vi "Sample_Finite_HardwareDelay.vi"() -> ()   [LabVIEW 2013]
doc: "This samples demonstrates how to sample a finite waveform."
uses:
  <userlib>/ArtScope/Trigger/ArtScope_ConfigureTriggerDigital.vi
  <userlib>/ArtScope/Fetch/ArtScope_FetchBinary16.vi
  <userlib>/ArtScope/_SubVI/ArtScope_ArrayByChannel_U16.vi
panel:
  out "error out":errorcluster
  in  "reference position":dbl
  in  "source":string(combo)="VAL_TRIGGER_DTR"
  in  "edge":i32(ring) items=["Negative", "Positive", "NegatiPosit"]
  in  "sensitive":i32=50
  in  "count":i32=1
  in  "range(Vpp)":i32(ring)=1 items=["20V", "10V", "2V", "40V", "16V", "8V", "4V", "1.6V", "800m", "400m", "160m", "80m", "40m"]
  in  "offset(mV)":i32
  in  "NumSamples":i32=1000
  in  "Stop":bool
  out "waveform":u16[][](graph)
  in  "Timeout(s)":dbl=10.0
  in  "MinRecordLength":i32=6000
  in  "MinSampleRate":dbl=800000.0
  in  "Coupling":i32(ring) items=["DC", "AC"]
  in  "Channel Name":string="0,1"
  in  "Resource Name":string="Dev1"
  # "Vertical"
  # "Horizontal"
  # "Trigger"
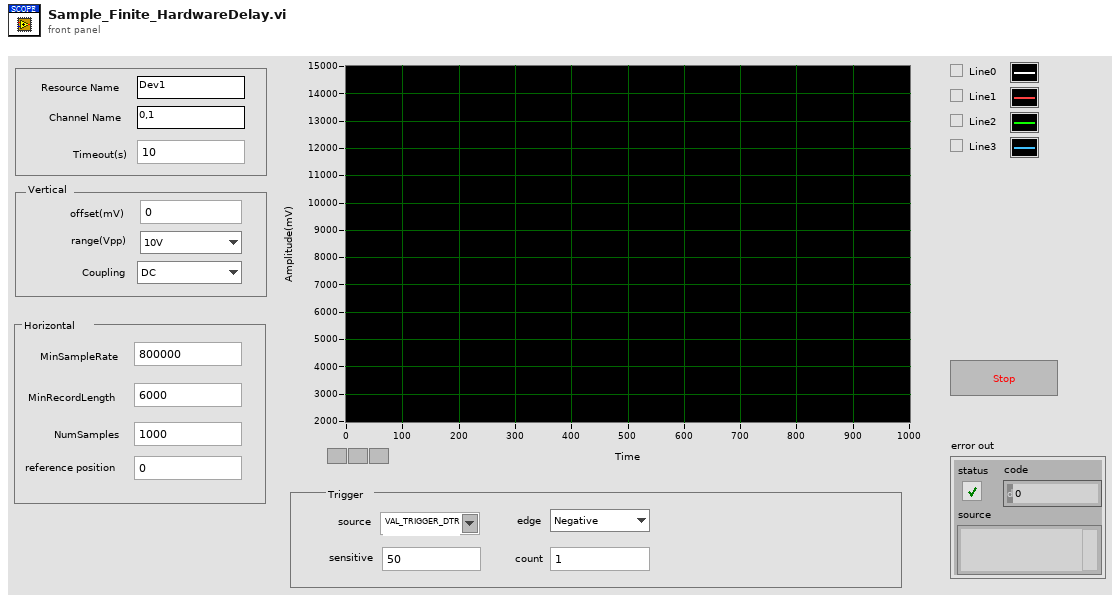
[diagram p1: front panel]
types:
  T1 = cluster{"fLSB":cluster{dbl, dbl, dbl, dbl, dbl, dbl, dbl, dbl}, "RangeValue":cluster{dbl, dbl, dbl, dbl, dbl, dbl, dbl, dbl}, "wMaxLSB":u32, "TriggerMode":i32, "sampLengthPerChan":u32, "pAvailSampsPoints":u32, "channelCount":i32}
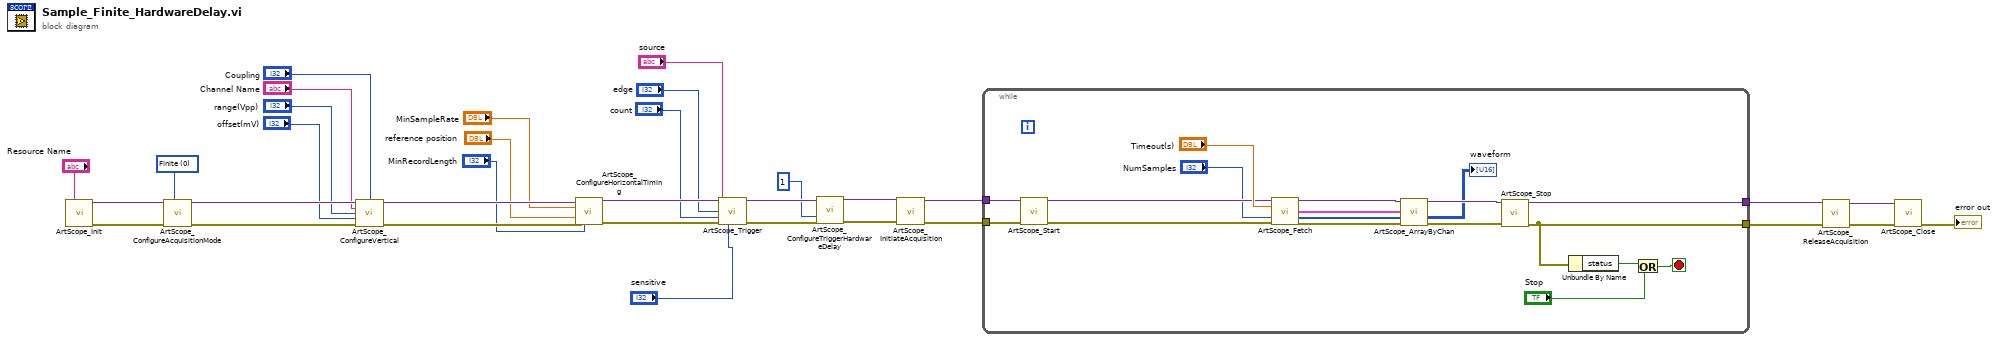
[diagram p0: block diagram]
diagram:
  w26 = 0 items=["Finite", "Continuous"] ("AcuqMode")
  n1 = call <userlib>:"ArtScope_Init.vi"("task name"="Resource Name") -> ("task handle"=w27:variant, "error out"=w28:errorcluster)  [unwired: 13 in]
  n2 = call <userlib>:"ArtScope_ConfigureAcquisitionMode.vi"("task handle"=w27, "acquisition mode"=w26, "error in (no error)"=w28) -> ("task handle"=w25:variant, "error out"=w29:errorcluster)  [unwired: 11 in]
  n3 = call <userlib>:"ArtScope_ConfigureVertical.vi"("task handle"=w25, "coupling"="Coupling", "channels"="Channel Name", "range(Vpp)"="range(Vpp)", "offset"="offset(mV)", "error in (no error)"=w29) -> ("task handle"=w31:variant, "error out"=w30:errorcluster)  [unwired: 8 in]
  n4 = call <userlib>:"ArtScope_ConfigureHorizontalTiming.vi"("task handle"=w31, "min sample rate"="MinSampleRate", "reference position"="reference position", "error in (no error)"=w30, "min record length"="MinRecordLength") -> ("task handle"=w23:variant, "error out"=w24:errorcluster)  [unwired: 9 in]
  n5 = call-poly <userlib>:"ArtScope_Trigger.vi"("task handle"=w23, "trigger source"="source", "edge"="edge", "trigger count"="count", "error in (no error)"=w24, "trigger sensitive"="sensitive") -> ("task handle"=w6:variant, "error out"=w4:errorcluster)  [unwired: 8 in]
  n6 = call <userlib>:"ArtScope_ConfigureTriggerHardwareDelay.vi"("task handle"=w6, "delay points"=1, "error in (no error)"=w4) -> ("task handle"=w5:variant, "error out"=w3:errorcluster)  [unwired: 11 in]
  n7 = call <userlib>:"ArtScope_InitiateAcquisition.vi"("task handle"=w5, "error in (no error)"=w3) -> ("task handle"=w15:variant, "error out"=w14:errorcluster)  [unwired: 12 in]
  n8 = while {
    tunnel: [w47] -> w19
    tunnel: [w46] -> w18
    tunnel: w15 -> [w45]
    tunnel: w14 -> [w50]
    stop <- w48 stop-if-true
    n9 = call <userlib>:"ArtScope_Start.vi"("task handle"=w45, "error in (no error)"=w50) -> ("task handle"=w43:variant, "error out"=w42:errorcluster)  [unwired: 12 in]
    n10 = call-poly <userlib>:"ArtScope_Fetch.vi"("task handle"=w43, "timeout"="Timeout(s)", "num samples"="NumSamples", "error in (no error)"=w42) -> ("task handle"=w40:variant, "wfm info"=w36:T1, "data"=w35:u16[], "error out"=w37:errorcluster)  [unwired: 8 in]
    n11 = call-poly <userlib>:"ArtScope_ArrayByChan.vi"("task handle"=w40, "wfm info"=w36, "1D data"=w35, "error in (no error)"=w37) -> ("task handle"=w39:variant, "2D data"=→"waveform":u16[][], "error out"=w38:errorcluster)  [unwired: 9 in]
    n12 = call <userlib>:"ArtScope_Stop.vi"("task handle"=w39, "error in (no error)"=w38) -> ("task handle"=w47:variant, "error out"=w46:errorcluster)  [unwired: 12 in]
    n13 = Unbundle By Name(w46) -> ("status"=w49:bool)
    n14 = Or(x=w49, y="Stop") -> (x .or. y?=w48:bool)
  }
  n15 = call <userlib>:"ArtScope_ReleaseAcquisition.vi"("task handle"=w19, "error in (no error)"=w18) -> ("task handle"=w17:variant, "error out"=w16:errorcluster)  [unwired: 12 in]
  n16 = call <userlib>:"ArtScope_Close.vi"("task handle"=w17, "error in (no error)"=w16) -> ("error out"=→"error out":errorcluster)  [unwired: 13 in]
